vi "WLAN Dut Tx Configure.vi"(0 "niDTS WLAN DUT in":refnum<class "niDTS WLAN Dut.lvclass">, 11 "error in (no error)":errorcluster) -> (4 "niDTS WLAN DUT out":refnum<class "niDTS WLAN Dut.lvclass">, 15 "error out":errorcluster)   [LabVIEW 2015, in "niDTS WLAN.lvlib" / "niDTS WLAN Dut.lvclass"]
uses:
  niDTS WLAN Dut.lvclass
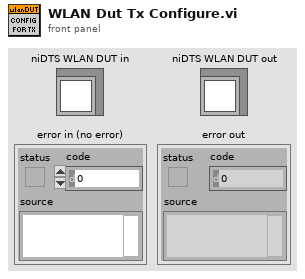
[diagram p1: front panel]
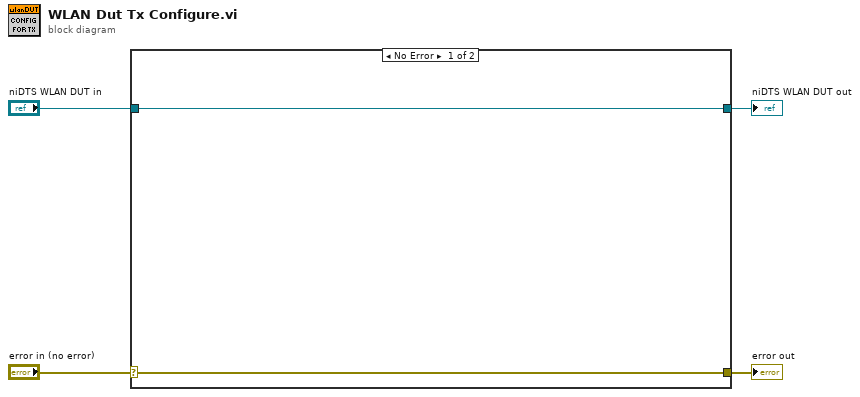
[diagram p0: block diagram]
diagram:
  n1 = case shown="No Error" "error in (no error)" {
    selector: "error in (no error)" -> [w5 w8]
    tunnel: [w5 w8] -> w3
    tunnel: [w6 w7] -> w1
    tunnel: "niDTS WLAN DUT in" -> [w6 w7]
    frame No Error {
    }
    frame Error {
    }
  }
  "error out" <- w3
  "niDTS WLAN DUT out" <- w1
